vi "Vec2MPOR.vi"(8 "SignalName":string, 9 "ClusterSigFormat":T1, 10 "格式":string, 11 "DataIn":u32[](array[numeric])) -> (1 "isTrue":bool, 3 "MPOR":i32)   [LabVIEW 2015]
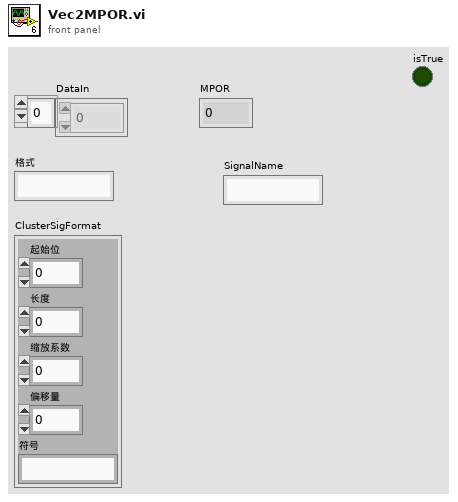
[diagram p1: front panel]
types:
  T1 = cluster{"起始位":u8, "长度":u8, "缩放系数":dbl, "偏移量":dbl, "符号":string}
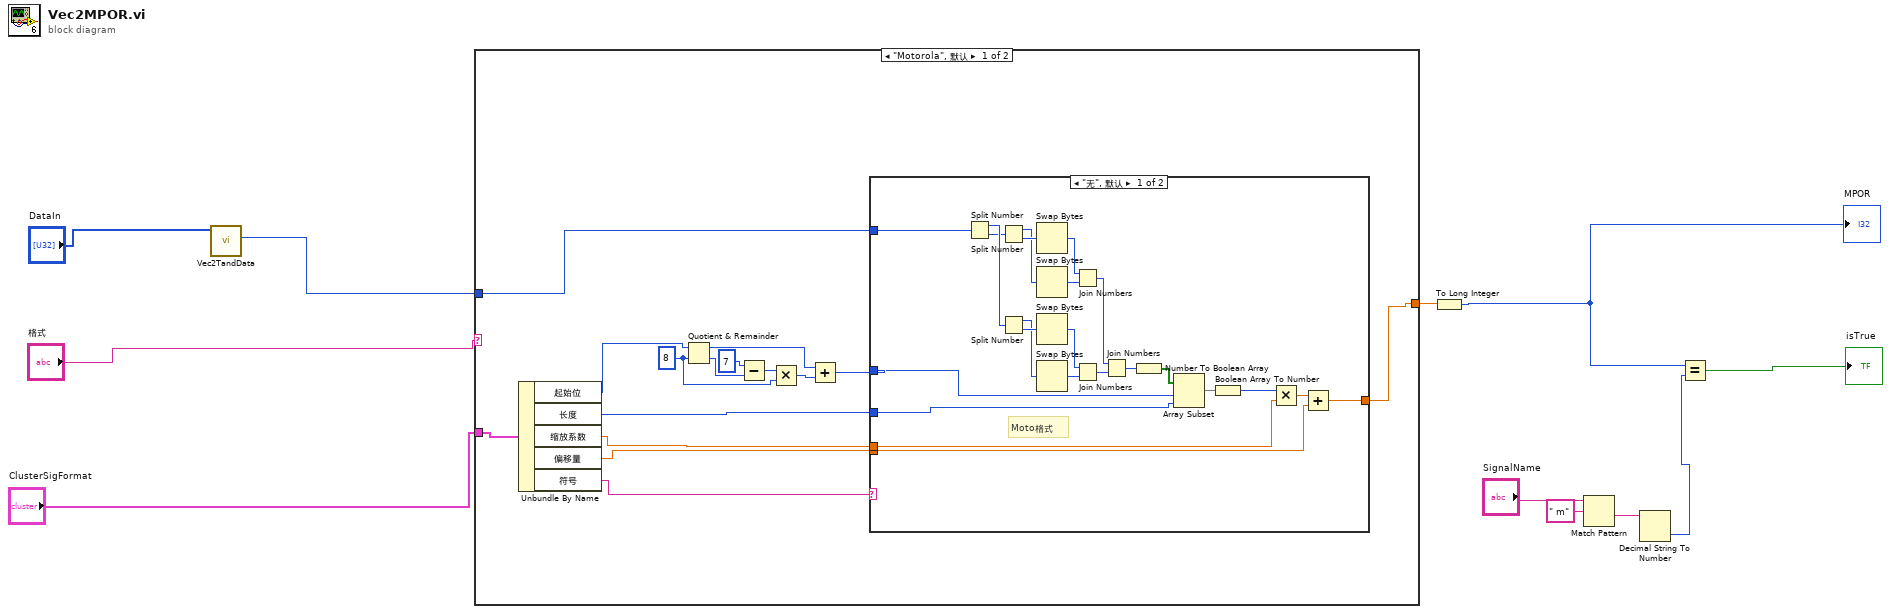
[diagram p0: block diagram]
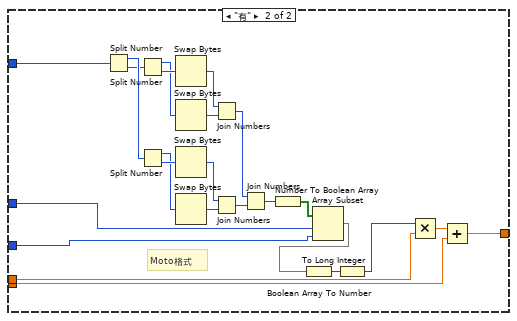
[diagram p2: hidden frame]
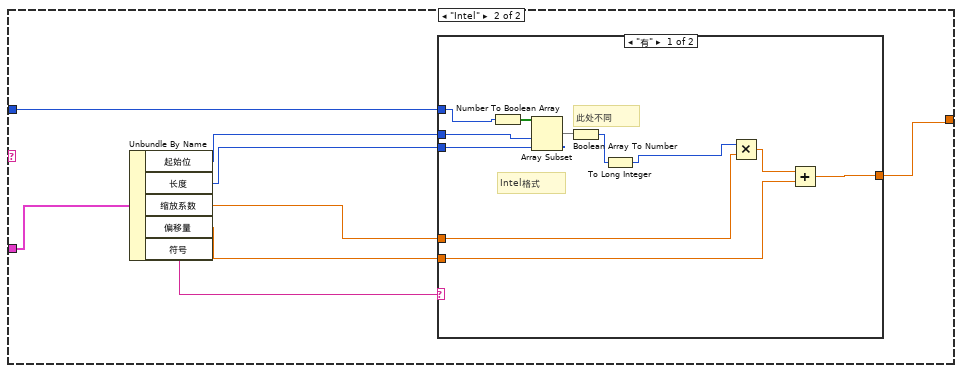
[diagram p3: hidden frame]
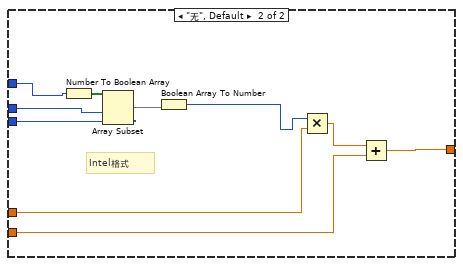
[diagram p4: hidden frame]
diagram:
  n1 = call "Vec2TandData.vi"("Frames"="DataIn") -> ("_64Bits"=w8:u64)  [unwired: 9 in, 1 out]
  n2 = case shown="\"Motorola\", 默认" "格式" {
    tunnel: "ClusterSigFormat" -> [w14 w75]
    tunnel: w8 -> [w13 w76]
    tunnel: [w12 w74] -> w7
    frame "Motorola", Default {
      w21 = 8
      n3 = Unbundle By Name(w14) -> ("起始位"=w16:u8, "长度"=w17:u8, "缩放系数"=w18:dbl, "偏移量"=w19:dbl, "符号"=w15:string)
      n4 = Quotient & Remainder(x=w16, y=w21) -> (x-y*floor(x/y)=w26:i32, floor(x/y)=w24:i32)
      n5 = Subtract(x=7, y=w24) -> (x-y=w25:i32)
      n6 = Multiply(x=w25, y=w21) -> (x*y=w23:i32)
      n7 = Add(x=w26, y=w23) -> (x+y=w20:i32)
      n8 = case shown="\"无\", 默认" w15 {
        tunnel: [w49 w73] -> w12
        tunnel: w20 -> [w46 w70]
        tunnel: w13 -> [w45 w69]
        tunnel: w19 -> [w44 w68]
        tunnel: w18 -> [w43 w67]
        tunnel: w17 -> [w42 w66]
        frame "无", Default {
          # "Moto格式"
          n9 = Split Number(x=w45) -> (hi(x)=w40:u32, lo(x)=w39:u32)
          n10 = Split Number(x=w39) -> (hi(x)=w37:u16, lo(x)=w38:u16)
          n11 = Split Number(x=w40) -> (hi(x)=w35:u16, lo(x)=w36:u16)
          n12 = Swap Bytes(anything=w38) -> (byte swapped=w32:u16)
          n13 = Swap Bytes(anything=w37) -> (byte swapped=w31:u16)
          n14 = Swap Bytes(anything=w36) -> (byte swapped=w33:u16)
          n15 = Swap Bytes(anything=w35) -> (byte swapped=w34:u16)
          n16 = Join Numbers(hi=w32, lo=w31) -> ((hi.lo)=w29:u32)
          n17 = Join Numbers(hi=w33, lo=w34) -> ((hi.lo)=w30:u32)
          n18 = Join Numbers(hi=w29, lo=w30) -> ((hi.lo)=w28:u64)
          n19 = Number To Boolean Array(number=w28) -> (Boolean array=w27:bool[])
          n20 = Array Subset(array=w27, index=w46, length=w42) -> (w41:bool[])
          n21 = Boolean Array To Number(Boolean array=w41) -> (number=w47:u32)
          n22 = Multiply(x=w47, y=w43) -> (x*y=w48:dbl)
          n23 = Add(x=w48, y=w44) -> (x+y=w49:dbl)
        }
        frame "有" {
          # "Moto格式"
          n24 = Split Number(x=w69) -> (hi(x)=w64:u32, lo(x)=w63:u32)
          n25 = Split Number(x=w63) -> (hi(x)=w61:u16, lo(x)=w62:u16)
          n26 = Split Number(x=w64) -> (hi(x)=w59:u16, lo(x)=w60:u16)
          n27 = Swap Bytes(anything=w62) -> (byte swapped=w56:u16)
          n28 = Swap Bytes(anything=w61) -> (byte swapped=w55:u16)
          n29 = Swap Bytes(anything=w60) -> (byte swapped=w57:u16)
          n30 = Swap Bytes(anything=w59) -> (byte swapped=w58:u16)
          n31 = Join Numbers(hi=w56, lo=w55) -> ((hi.lo)=w53:u32)
          n32 = Join Numbers(hi=w57, lo=w58) -> ((hi.lo)=w54:u32)
          n33 = Join Numbers(hi=w53, lo=w54) -> ((hi.lo)=w52:u64)
          n34 = Number To Boolean Array(number=w52) -> (Boolean array=w51:bool[])
          n35 = Array Subset(array=w51, index=w70, length=w66) -> (w65:bool[])
          n36 = Boolean Array To Number(Boolean array=w65) -> (number=w50:u32)
          n37 = To Long Integer(number=w50) -> (32bit integer=w71:i32)
          n38 = Multiply(x=w71, y=w67) -> (x*y=w72:dbl)
          n39 = Add(x=w72, y=w68) -> (x+y=w73:dbl)
        }
      }
    }
    frame "Intel" {
      n40 = Unbundle By Name(w75) -> ("起始位"=w81:u8, "长度"=w80:u8, "缩放系数"=w79:dbl, "偏移量"=w78:dbl, "符号"=w77:string)
      n41 = case shown="\"有\"" w77 {
        tunnel: [w92 w102] -> w74
        tunnel: w81 -> [w89 w99]
        tunnel: w80 -> [w88 w98]
        tunnel: w79 -> [w87 w97]
        tunnel: w78 -> [w86 w96]
        tunnel: w76 -> [w82 w93]
        frame "有" {
          # "此处不同"
          # "Intel格式"
          n42 = Number To Boolean Array(number=w82) -> (Boolean array=w85:bool[])
          n43 = Array Subset(array=w85, index=w89, length=w88) -> (w84:bool[])
          n44 = Boolean Array To Number(Boolean array=w84) -> (number=w83:u32)
          n45 = To Long Integer(number=w83) -> (32bit integer=w90:i32)
          n46 = Multiply(x=w90, y=w87) -> (x*y=w91:dbl)
          n47 = Add(x=w91, y=w86) -> (x+y=w92:dbl)
        }
        frame "无", Default {
          # "Intel格式"
          n48 = Number To Boolean Array(number=w93) -> (Boolean array=w95:bool[])
          n49 = Array Subset(array=w95, index=w99, length=w98) -> (w94:bool[])
          n50 = Boolean Array To Number(Boolean array=w94) -> (number=w100:u32)
          n51 = Multiply(x=w100, y=w97) -> (x*y=w101:dbl)
          n52 = Add(x=w101, y=w96) -> (x+y=w102:dbl)
        }
      }
    }
  }
  n53 = To Long Integer(number=w7) -> (32bit integer=w2:i32)
  "MPOR" <- w2
  n54 = Match Pattern(string="SignalName", regular expression=" m" ("正则表达式")) -> (after substring=w4:string)  [unwired: 1 in, 3 out]
  n55 = Decimal String To Number(string=w4) -> (number=w3:i32)  [unwired: 2 in, 1 out]
  n56 = Equal?(x=w2, y=w3) -> (x = y?=→"isTrue":bool)
